vi "ReadXmlFile.vi"() -> ()   [LabVIEW 2016]
uses:
  <vilib>/Utility/xml.llb/Read From XML File(array).vi
  <vilib>/Utility/xml.llb/Read From XML File(string).vi
  <vilib>/xml/Load XML File.vi
  <vilib>/xml/NI_XML.lvlib
  <resource>/objmgr/DOMUserDefRef.rc
panel:
  out "Can Bus ID":string
  out "Debug Array 2":string[](array[string])
  out "Numeric 2":i32
  out "Numeric 1":i32
  out "node text":string
  out "Debug Array 1":string[](array[string])
  in  "Robot Id xPath":string="ControlDefinition/RobotId"
  out "Debug XML Array":string[](array[string])
  out "Debug XML String":string
  in  "file path (dialog if empty) 2":path=path "C:/git/ViTestFiles/RobotConfiguration-7.xml"
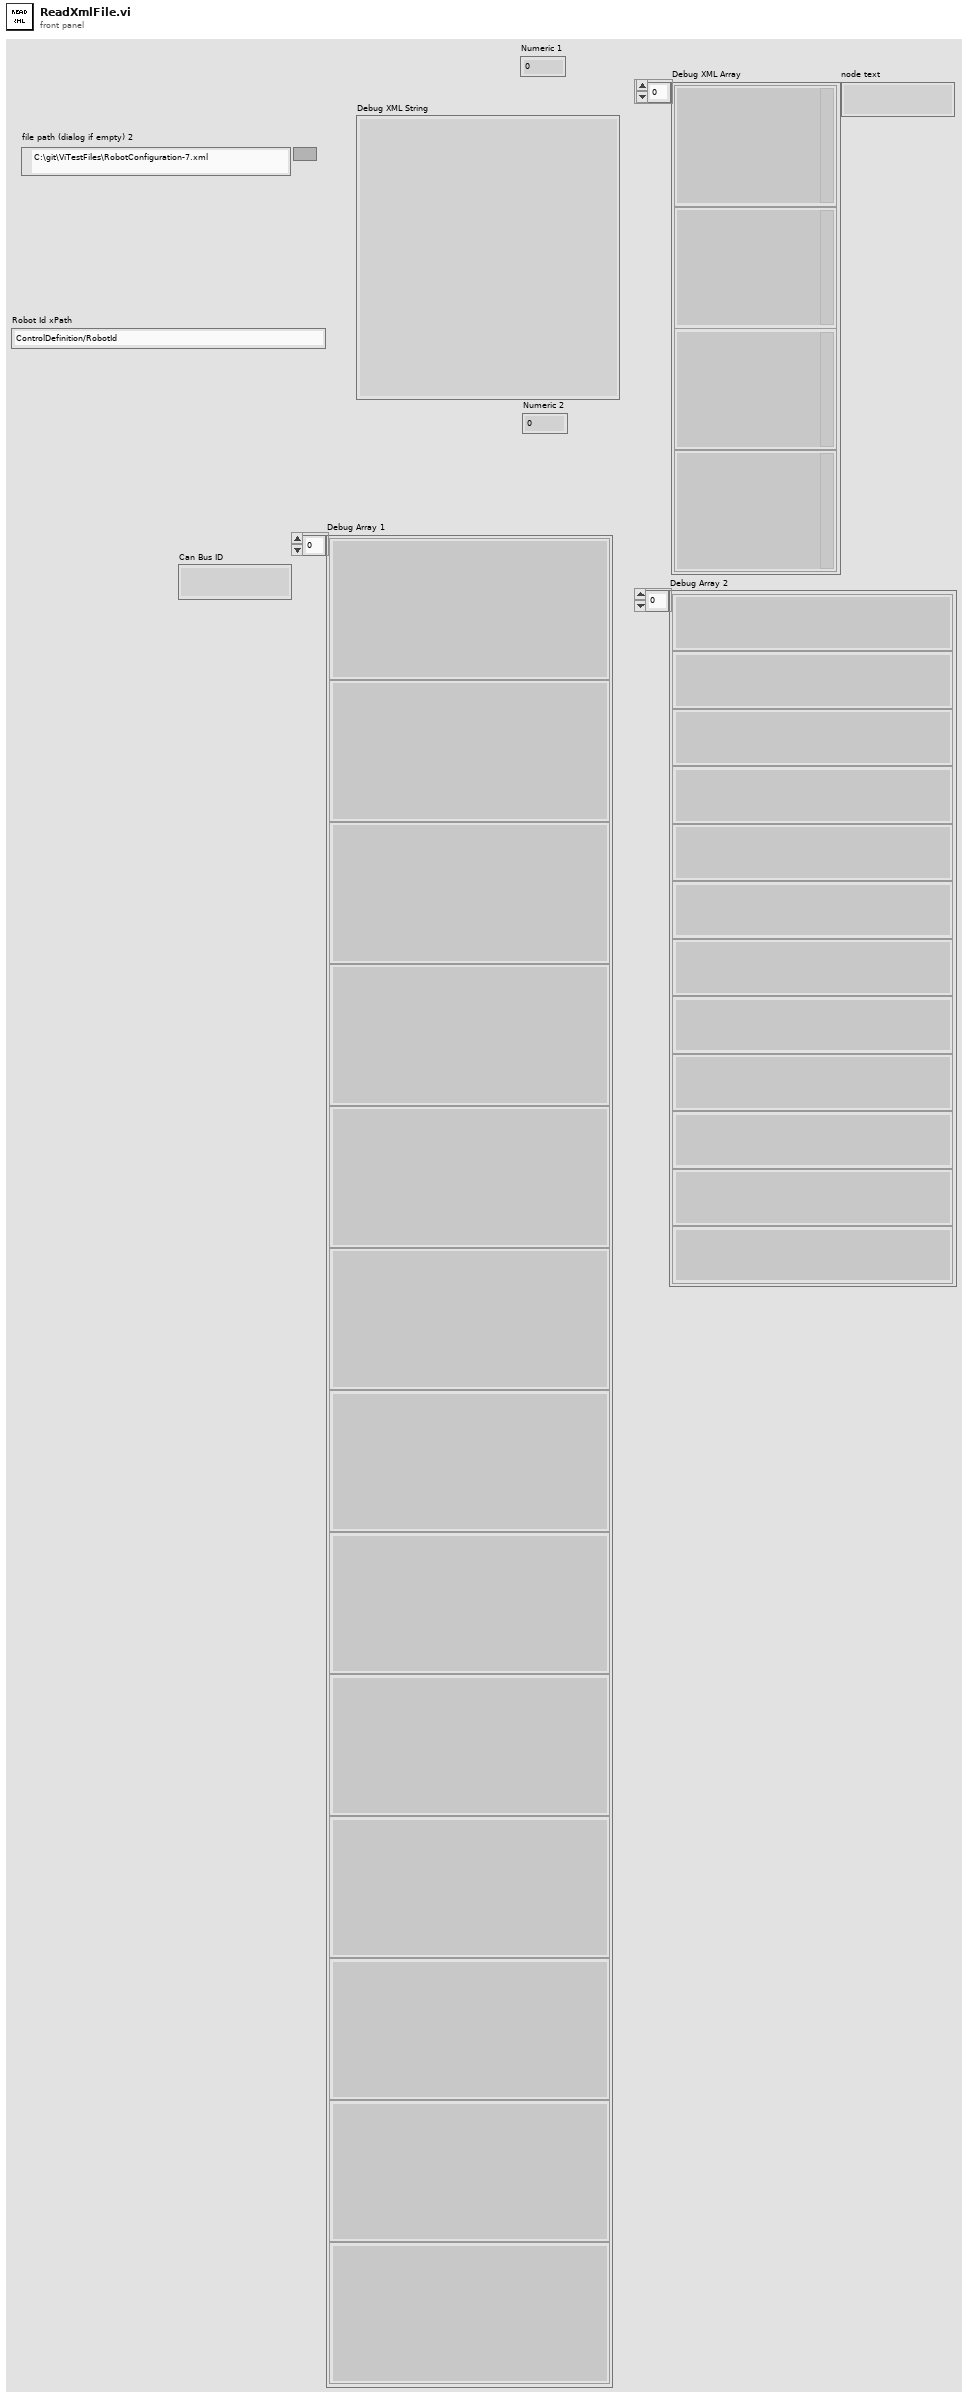
[diagram p1: front panel]
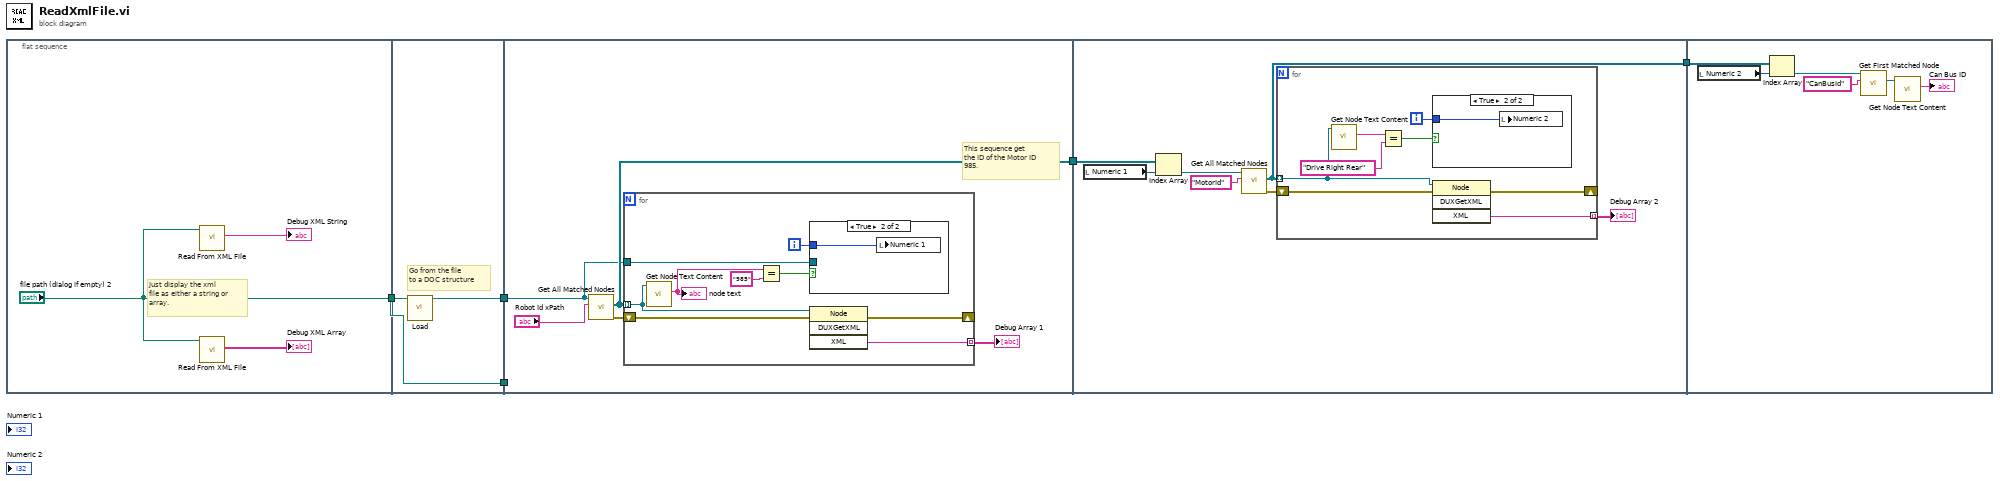
[diagram p0: block diagram]
diagram:
  n1 = flat-sequence {
    tunnel: ["file path (dialog if empty) 2"] -> w5
    tunnel: w5 -> [w10]
    tunnel: [w10] -> w4
    tunnel: [w9] -> w3
    tunnel: [w13] -> w2
    tunnel: w4 -> [_]
    tunnel: w3 -> [w11]
    tunnel: w2 -> [w30]
    tunnel: [w26] -> w1
    tunnel: w1 -> [w47]
    frame #0 {
      # "Just display the xml\nfile as either a string or\narray."
      n2 = call-poly <vilib>:"Read From XML File.vi"("XML File Path"="file path (dialog if empty) 2") -> ("XML Elements"=→"Debug XML String":string)  [unwired: 8 in, 2 out]
      n3 = call-poly <vilib>:"Read From XML File.vi"("XML File Path"="file path (dialog if empty) 2") -> ("XML Elements"=→"Debug XML Array":string[])  [unwired: 8 in, 2 out]
    }
    frame #1 {
      # "Go from the file\nto a DOC structure"
      n4 = call-poly <vilib>:"Load.vi"("path to XML document"=w10) -> ("DOM document out"=w9:refnum<k20>)  [unwired: 12 in, 2 out]
    }
    frame #2 {
      # "This sequence get\nthe ID of the Motor ID\n985."
      n5 = call <vilib>:"Get All Matched Nodes.vi"("XPath expression"="Robot Id xPath", "node in"=w11) -> ("error out"=w15:errorcluster, "node result array"=w13:refnum<k20>[])  [unwired: 7 in, 1 out]
      n6 = for {
        shift-right: [w22] -> _
        shift-left: w15 -> [w23]
        tunnel: [w24] -> w12 mode=indexing
        tunnel: w13 -> [w21] mode=indexing
        tunnel: w11 -> [w17]
        i -> [w16]
        n7 = call <vilib>:"Get Node Text Content.vi"("node in"=w21) -> ("node text"=w20:string)  [unwired: 8 in, 2 out]
        "node text" <- w20
        n8 = Equal?(x=w20, y="985") -> (x = y?=w18:bool)
        n9 = case shown="True" w18 {
          tunnel: w17 -> [_ _]
          tunnel: w16 -> [_ w25]
          frame False {
          }
          frame True {
            n10 = local write "Numeric 1"(w25) -> ()
          }
        }
        n11 = invoke on="Invoke Node" class="Node" method="DUXGetXML"(reference=w21, error in=w23) -> (error out=w22:errorcluster, "XML"=w24:string)  [unwired: 2 in, 2 out]
      }
      "Debug Array 1" <- w12
    }
    frame #3 {
      n12 = local read "Numeric 1"() -> (w32:i32)
      n13 = Index Array(array=w30, index=w32) -> (element=w29:refnum<k20>)
      n14 = call <vilib>:"Get All Matched Nodes.vi"("XPath expression"="MotorId" ("Motor Id xPath"), "node in"=w29) -> ("error out"=w28:errorcluster, "node result array"=w26:refnum<k20>[])  [unwired: 7 in, 1 out]
      n15 = for {
        shift-right: [w39] -> _
        shift-left: w28 -> [w40]
        tunnel: w26 -> [w34] mode=indexing
        tunnel: [w33] -> w27 mode=indexing
        i -> [w35]
        n16 = call <vilib>:"Get Node Text Content.vi"("node in"=w34) -> ("node text"=w38:string)  [unwired: 8 in, 2 out]
        n17 = Equal?(x=w38, y="Drive Right Rear") -> (x = y?=w36:bool)
        n18 = case shown="True" w36 {
          tunnel: w35 -> [_ w41]
          frame False {
          }
          frame True {
            n19 = local write "Numeric 2"(w41) -> ()
          }
        }
        n20 = invoke on="Invoke Node" class="Node" method="DUXGetXML"(reference=w34, error in=w40) -> (error out=w39:errorcluster, "XML"=w33:string)  [unwired: 2 in, 2 out]
      }
      "Debug Array 2" <- w27
    }
    frame #4 {
      n21 = local read "Numeric 2"() -> (w46:i32)
      n22 = Index Array(array=w47, index=w46) -> (element=w45:refnum<k20>)
      n23 = call <vilib>:"Get First Matched Node.vi"("XPath expression"="CanBusId", "node in"=w45) -> ("node result"=w43:refnum<k20>)  [unwired: 7 in, 2 out]
      n24 = call <vilib>:"Get Node Text Content.vi"("node in"=w43) -> ("node text"=→"Can Bus ID":string)  [unwired: 8 in, 2 out]
    }
  }
